vi "ConvertScanSourceToString.vi"(11 "Scan Source":T1=enum."Immediate") -> (3 "String":string)   [LabVIEW 2012, in "Keithley-7001.lvlib"]
uses:
  Keithley-7001.lvlib
  Public/Controls/ScanSource.ctl
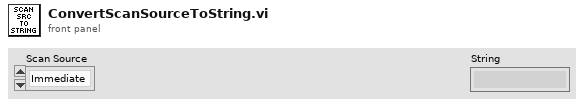
[diagram p1: front panel]
types:
  T1 = typedef "Keithley-7001.lvlib/ScanSource.ctl" = enum16{"Hold", "Immediate", "Timer", "Manual", "Bus", "TLink", "External"}
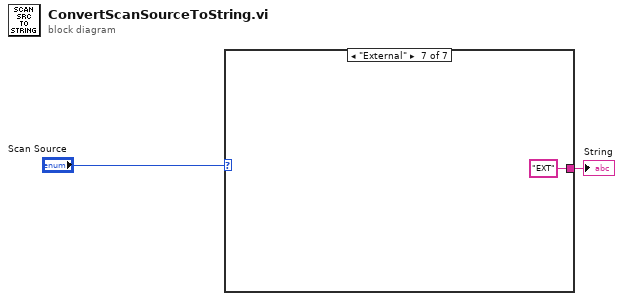
[diagram p0: block diagram]
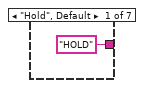
[diagram p2: hidden frame]
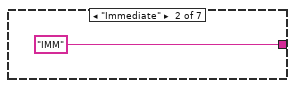
[diagram p3: hidden frame]
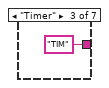
[diagram p4: hidden frame]
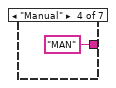
[diagram p5: hidden frame]
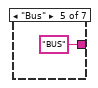
[diagram p6: hidden frame]
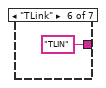
[diagram p7: hidden frame]
diagram:
  n1 = case shown="\"External\"" "Scan Source" {
    tunnel: ["HOLD" "IMM" "TIM" "MAN" "BUS" "TLIN" "EXT"] -> w1
    frame "Hold", Default {
    }
    frame "Immediate" {
    }
    frame "Timer" {
    }
    frame "Manual" {
    }
    frame "Bus" {
    }
    frame "TLink" {
    }
    frame "External" {
    }
  }
  "String" <- w1
